vi "Do Core.vi"(8 "error in (no error)":errorcluster caption="错误输入（无错误）", 9 "Actor in":refnum<class "Actor.lvclass"> caption="操作者输入", 11 "Reply Message":refnum<class "读取发送事件引用消息.lvclass"> caption="回复消息") -> (0 "error out":errorcluster caption="错误输出", 1 "Actor out":refnum<class "Actor.lvclass"> caption="操作者输出", 2 "Reply":variant caption="回复")   [LabVIEW 2015, in "上位机.lvlib" / "读取发送事件引用消息.lvclass"]
doc: "(<B>Filename</B>: Actor Framework.lvlib:Reply Msg.lvclass:Do Core.vi)\n\nDefines what an actor does when it receives <B>Reply Message</B>. This method also defines the <B>Reply</B> that is returned to the actor that sent <B>Reply Message</B>.\n\nBy default, this method does nothing, and <B>Reply</B> is the ancestor Message class. A child class must override this method to define behavior and specify a child of the Message class to return in the <B>Reply</B> output."
uses:
  <vilib>/ActorFramework/Actor/Actor.lvclass
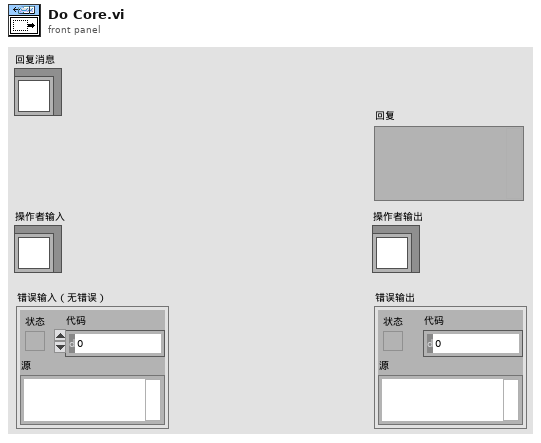
[diagram p1: front panel]
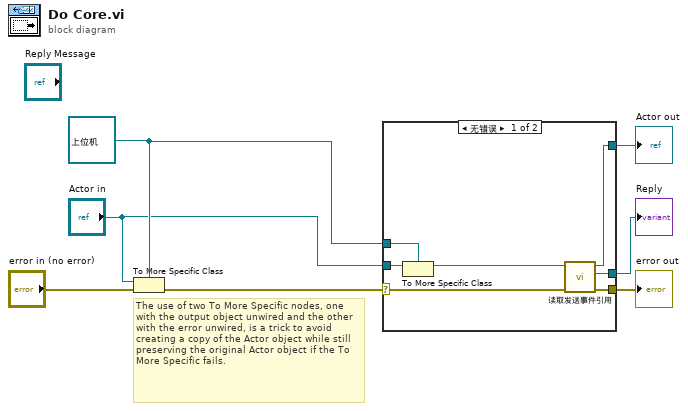
[diagram p0: block diagram]
diagram:
  w6 = refnum<class "上位机.lvclass"> refnum ("Actor in")
  # "The use of two To More Specific nodes, one with the output object unwired and the other with the error unwired, is a trick to avoid creating a copy of the Actor object while still preserving the original Actor object if the To More Specific fails."
  n1 = To More Specific Class(target class=w6, reference="Actor in", error in="error in (no error)") -> (error out=w7:errorcluster)  [unwired: 1 out]
  n2 = case shown="无错误" w7 {
    selector: w7 -> [w12 w16]
    tunnel: [w14 w16] -> w1
    tunnel: [w13 w15] -> w2
    tunnel: "Actor in" -> [w11 w15]
    tunnel: w6 -> [w10 _]
    tunnel: [w8 _] -> w3
    frame No Error {
      n3 = To More Specific Class(target class=w10, reference=w11) -> (specific class reference=w9:refnum<class "上位机.lvclass">)  [unwired: 1 in, 1 out]
      n4 = call "读取发送事件引用.vi"("error in (no error)"=w12, "上位机 输入"=w9) -> ("error out"=w14:errorcluster, "发送数据用户事件"=w8:refnum<user-event>, "上位机 输出"=w13:refnum<class "上位机.lvclass">)  [unwired: 7 in]
    }
    frame Error {
      # "If type check fails, pass the original object out again."
    }
  }
  "error out" <- w1
  "Actor out" <- w2
  "Reply" <- w3
